vi "PID.vi"(7 "PID gains":T1={"proportional gain (Kc)"=1.0, "integral time (Ti, min)"=0.01, "derivative time (Td, min)"=0.0} {"derivative time (Td, min)" format="%.3f"; "integral time (Ti, min)" format="%.3f"; "proportional gain (Kc)" format="%.3f"}, 8 "current theta1":dbl, 9 "current theta0":dbl, 10 "Des theta1":dbl, 11 "Des theta0":dbl) -> (0 "Dir2":bool, 1 "Dir1":bool, 2 "U2":dbl, 3 "U1":dbl)   [LabVIEW 2016, in "controllerLibrary.lvlib"]
uses:
  controllerLibrary.lvlib
  <vilib>/addons/control/pid/pid.llb/PID (DBL).vi
  <vilib>/addons/control/pid/NI_PID_pid.lvlib
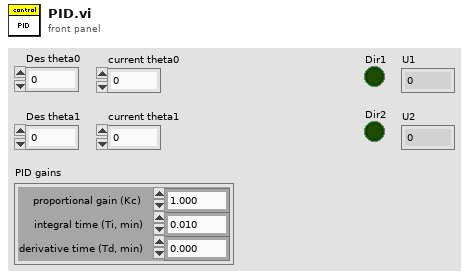
[diagram p1: front panel]
types:
  T1 = cluster{"proportional gain (Kc)":dbl, "integral time (Ti, min)":dbl, "derivative time (Td, min)":dbl}
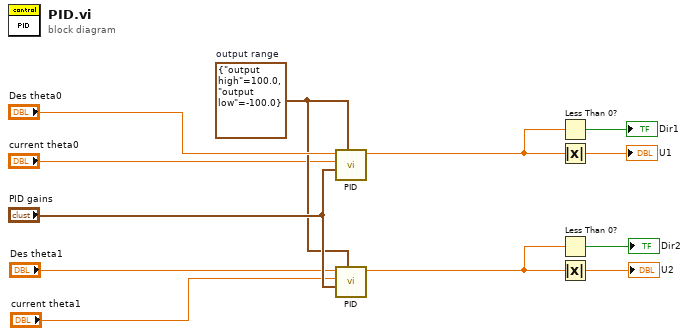
[diagram p0: block diagram]
diagram:
  w9 = cluster{"output high":dbl, "output low":dbl} {"output high"=100.0, "output low"=-100.0}  # output range
  n1 = call-poly <vilib>:"PID.vi"("output range"=w9, "PID gains"="PID gains", "process variable"="current theta0", "setpoint"="Des theta0") -> ("output"=w5:dbl)  [unwired: 6 in, 1 out]
  n2 = call-poly <vilib>:"PID.vi"("output range"=w9, "PID gains"="PID gains", "process variable"="current theta1", "setpoint"="Des theta1") -> ("output"=w3:dbl)  [unwired: 6 in, 1 out]
  n3 = Less Than 0?(x=w5) -> (x < 0?=→"Dir1":bool)
  n4 = Absolute Value(x=w5) -> (abs(x)=→"U1":dbl)
  n5 = Less Than 0?(x=w3) -> (x < 0?=→"Dir2":bool)
  n6 = Absolute Value(x=w3) -> (abs(x)=→"U2":dbl)
